vi "Task Setpoint Updated.vi"(7 "Task Ident":string, 8 "error in":errorcluster, 9 "Data":variant, 10 "Setpoint Ident":string, 11 "Series Actor in":refnum<class "Series Actor.lvclass">) -> (0 "error out":errorcluster, 3 "Series Actor out":refnum<class "Series Actor.lvclass">)   [LabVIEW 2024, in "Series Actor.lvlib" / "Series Actor.lvclass"]
uses:
  Series Actor.lvclass
  Series Actor.lvclass/Series Actor.ctl
  ISeries UI Actor/ISeries UI Actor Messages/Point Data Updated Msg/Update Point Data Msg.lvclass/Update Point Data Msg.ctl
  <vilib>/ActorFramework/Message Enqueuer/Message Enqueuer.lvclass/Message Enqueuer.ctl
  <vilib>/ActorFramework/Message Enqueuer/Enqueue.vi
  ISeries UI Actor/ISeries UI Actor Messages/Point Data Updated Msg/Update Point Data Msg.lvclass
  <vilib>/Utility/LVClass/Get LV Class Name.vi
  <resource>/AFDebug/Generate Trace for Message.vi
  <vilib>/ActorFramework/Message Priority Queue/Priority Enqueue.vi
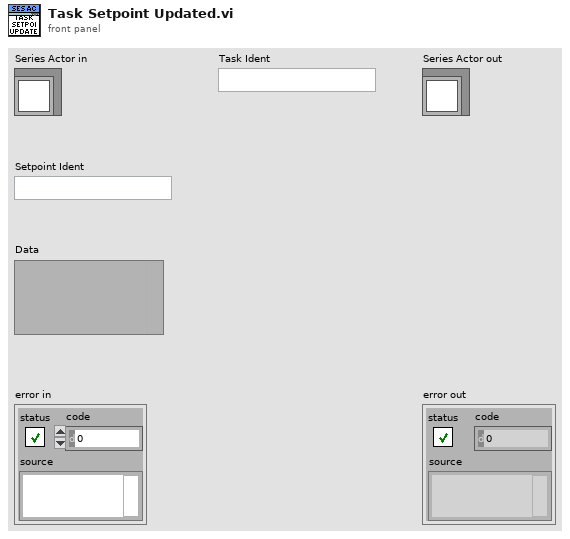
[diagram p1: front panel]
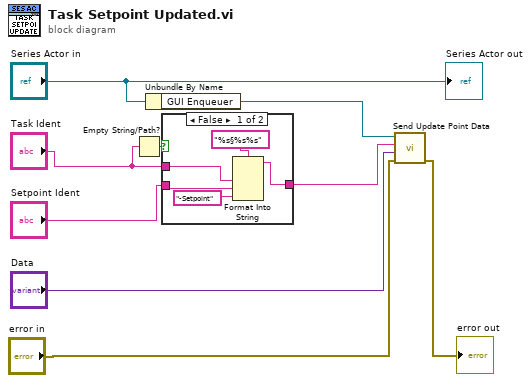
[diagram p0: block diagram]
diagram:
  n1 = Empty String/Path?(string/path="Task Ident") -> (empty?=w4:bool)
  n2 = Unbundle By Name("Series Actor in") -> ("GUI Enqueuer"=w8:refnum<class "Message Enqueuer.lvclass">)
  n3 = case shown="False" w4 {
    tunnel: "Task Ident" -> [w13 _]
    tunnel: "Setpoint Ident" -> [w12 w15]
    tunnel: [w11 w15] -> w1
    frame False {
      n4 = Format Into String(format string="%s§%s%s", w13, w12, "-Setpoint" ("input 3")) -> (resulting string=w11:string)  [unwired: 2 in, 1 out]
    }
    frame True {
    }
  }
  n5 = call "Send Update Point Data.vi"("error in (no error)"="error in", "Data"="Data", "Task-Point Ident"=w1, "Message Enqueuer"=w8) -> ("error out"=→"error out":errorcluster)  [unwired: 6 in, 1 out]
  "Series Actor out" <- "Series Actor in"
